vi "Goniometer_InterpolateData.vi"(8 "Input":dbl, 11 "Path":path) -> (2 "Output":dbl)   [LabVIEW 2018]
uses:
  <vilib>/Utility/file.llb/Read Delimited Spreadsheet (DBL).vi
  <vilib>/gmath/NI_Gmath.lvlib
panel:
  out "Angle (deg)":dbl[](array[numeric])
  out "Voltage (mV)":dbl[](array[numeric])
  out "Interpolated Angle (deg)":dbl[](array[numeric]) format="%_6g"
  # "Calibration Values"
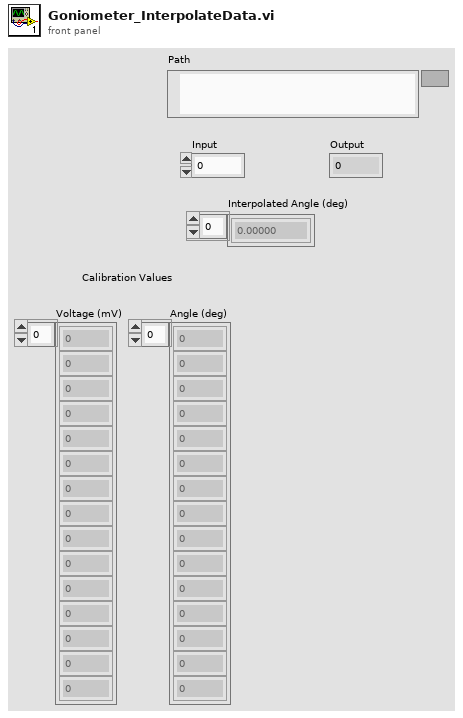
[diagram p1: front panel]
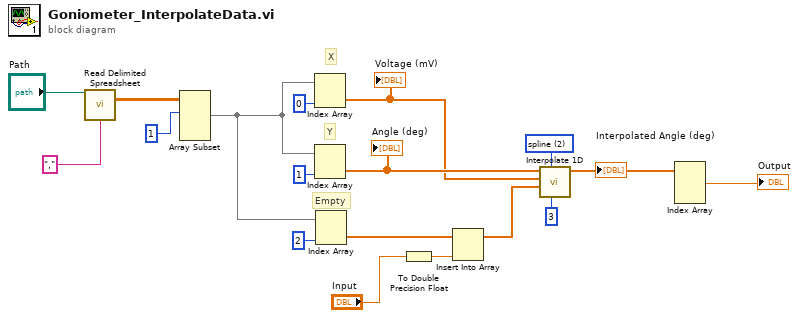
[diagram p0: block diagram]
diagram:
  w13 = 2 items=["nearest", "linear", "spline", "cubic Hermite", "Lagrange"] ("method")
  # "Empty"
  # "X"
  # "Y"
  n1 = call-poly <vilib>:"Read Delimited Spreadsheet.vi"("file path (dialog if empty)"="Path", "delimiter (\\t)"="," ("delimiter (\\t)")) -> ("all rows"=w16:dbl[][])  [unwired: 8 in, 5 out]
  n2 = Array Subset(array=w16, index (row)=1 ("index")) -> (w9:dbl[][])  [unwired: 3 in]
  n3 = Index Array(array=w9, index (col)=0 ("disabled index (col)")) -> (element=w10:dbl[])  [unwired: 1 in]
  "Voltage (mV)" <- w10
  n4 = Index Array(array=w9, index (col)=1 ("disabled index (col)")) -> (element=w11:dbl[])  [unwired: 1 in]
  "Angle (deg)" <- w11
  n5 = Index Array(array=w9, index (col)=2 ("disabled index (col)")) -> (element=w7:dbl[])  [unwired: 1 in]
  n6 = To Double Precision Float(number="Input") -> (double precision float=w6:dbl)
  n7 = Insert Into Array(array=w7, new element=w6) -> (w5:dbl[])  [unwired: 1 in]
  n8 = call <vilib>:"Interpolate 1D.vi"("ntimes"=3, "method"=w13, "xi"=w5, "X"=w10, "Y"=w11) -> ("yi"=w4:dbl[])  [unwired: 4 in, 2 out]
  "Interpolated Angle (deg)" <- w4
  n9 = Index Array(array=w4) -> (element #1=→"Output":dbl)  [unwired: 3 in, 2 out]
